vi "SUB_WriteMAC_toFile.vi"(2 "MAC Address":string) -> ()   [LabVIEW 2011]
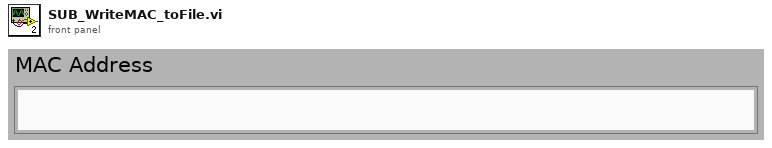
[diagram p1: front panel]
types:
  T1 = enum32{"invalid app kind", "Development System", "Run Time System", "Student Edition", "Embedded LabVIEW", "Evaluation", "Custom"}
  T2 = enum16{"open", "replace", "create", "open or create", "replace or create", "replace or create with confirmation"}
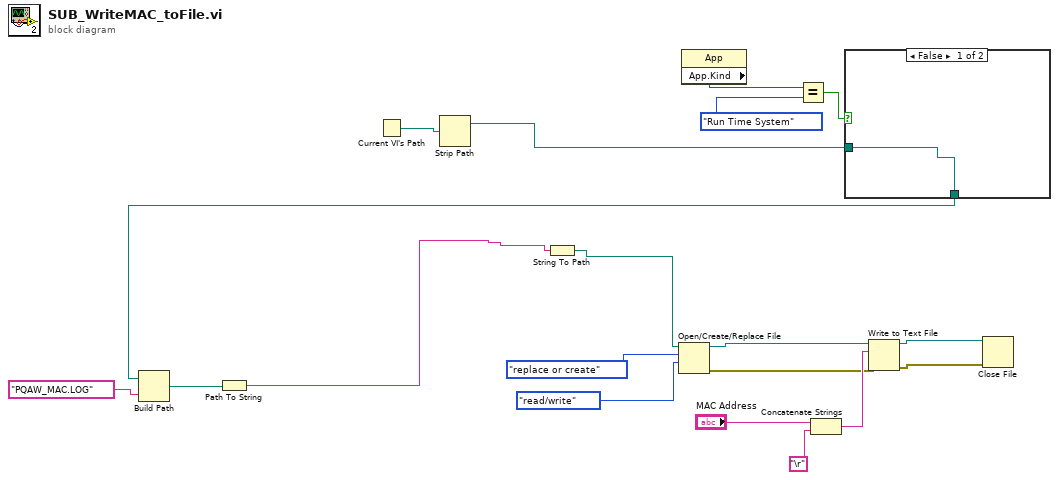
[diagram p0: block diagram]
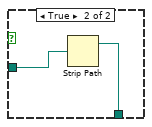
[diagram p2: hidden frame]
diagram:
  n1 = Current VI's Path() -> (path=w11:path)
  n2 = Strip Path(path=w11) -> (stripped path=w7:path)  [unwired: 1 out]
  n3 = property class="App"() -> ("App.Kind"=w10:T1)  [unwired: 2 in, 2 out]
  n4 = Equal?(x=w10, y=T1."Run Time System" ("Application:Kind")) -> (x = y?=w8:bool)
  n5 = Concatenate Strings("MAC Address", "\r") -> (w16:string)
  n6 = case shown="False" w8 {
    tunnel: w7 -> [w20 w22]
    tunnel: [w20 w21] -> w2
    frame False {
    }
    frame True {
      n7 = Strip Path(path=w22) -> (stripped path=w21:path)  [unwired: 1 out]
    }
  }
  n8 = Build Path(base path=w2, name or relative path="PQAW_MAC.LOG" ("string")) -> (appended path=w4:path)
  n9 = Path To String(path=w4) -> (string=w1:string)
  n10 = String To Path(string=w1) -> (path=w6:path)
  n11 = Open/Create/Replace File(file path (use dialog)=w6, operation (0:open)=T2."replace or create", access (0:read/write)=enum16{"read/write", "read-only", "write-only"}."read/write") -> (refnum out=w15:refnum<file>, error out=w5:errorcluster)  [unwired: 3 in, 1 out]
  n12 = Write to Text File(file (use dialog)=w15, text=w16, error in=w5) -> (refnum out=w13:refnum<file>, error out=w14:errorcluster)  [unwired: 1 in, 1 out]
  n13 = Close File(refnum=w13, error in=w14) -> ()  [unwired: 2 out]
